vi "From JSON.vi"(8 "error in (no error)":errorcluster, 11 "JSON":string) -> (0 "error out":errorcluster, 3 "Package out":refnum<class "Package.lvclass">)   [LabVIEW 2020, in "GCentral-API.lvlib" / "Package.lvclass"]
uses:
  Package.lvclass
  Package.lvclass/Package.ctl
  neg-pkg/JSON/JSON.lvlib
  Version/Version.lvclass
  Developer Group/Developer Group.lvclass
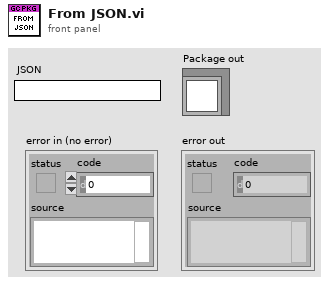
[diagram p1: front panel]
types:
  T1 = typedef "JSON.lvlib/JSON Item Type.ctl" = enum16{"unknown", "null", "Array", "Object", "String", "Number", "Boolean"}
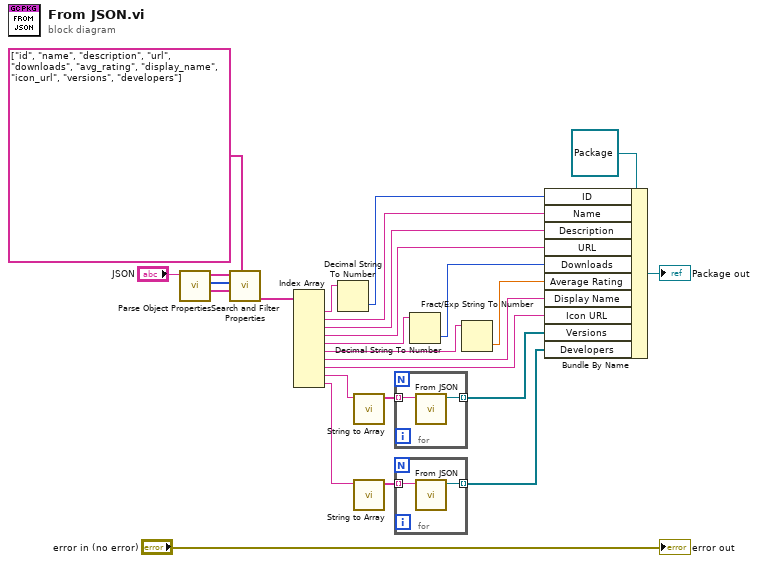
[diagram p0: block diagram]
diagram:
  n1 = call "Parse Object Properties.vi"("JSON String"="JSON") -> ("Values"=w20:string[], "Item Types"=w21:T1[], "Keys"=w22:string[])  [unwired: 7 in, 1 out]
  n2 = call "Search and Filter Properties.vi"("Search Keys"=string[] ["id", "name", "description", "url", "downloads", "avg_rating", "display_name", "icon_url", "versions", "developers"], "Values In"=w20, "Types In"=w21, "Keys In"=w22) -> ("Filtered Values"=w1:string[])  [unwired: 2 in, 5 out]
  n3 = Index Array(array=w1) -> (element #1=w18:string, element #2=w16:string, element #3=w15:string, element #4=w14:string, element #5=w13:string, element #6=w11:string, element #7=w9:string, element #8=w8:string, element #9=w7:string, element #10=w6:string)  [unwired: 10 in]
  n4 = Decimal String To Number(string=w18) -> (number=w17:i32)  [unwired: 2 in, 1 out]
  n5 = call "String to Array.vi"("Array String In"=w7) -> ("JSON Strings"=w5:string[])  [unwired: 10 in]
  n6 = call "String to Array.vi"("Array String In"=w6) -> ("JSON Strings"=w3:string[])  [unwired: 10 in]
  n7 = for {
    tunnel: w5 -> [w28] mode=indexing
    tunnel: [w27] -> w4 mode=indexing
    n8 = call "From JSON.vi"("JSON"=w28) -> ("Version"=w27:refnum<class "Version.lvclass">)  [unwired: 9 in, 1 out]
  }
  n9 = for {
    tunnel: w3 -> [w30] mode=indexing
    tunnel: [w29] -> w2 mode=indexing
    n10 = call "From JSON.vi"("JSON"=w30) -> ("Developer Group out"=w29:refnum<class "Developer Group.lvclass">)  [unwired: 9 in, 1 out]
  }
  n11 = Decimal String To Number(string=w13) -> (number=w12:i32)  [unwired: 2 in, 1 out]
  n12 = Fract/Exp String To Number(string=w11) -> (number=w10:dbl)  [unwired: 3 in, 1 out]
  n13 = Bundle By Name(cluster=refnum<class "Package.lvclass"> refnum ("GCentral-API.lvlib:Package.lvclass"), "ID"=w17, "Name"=w16, "Description"=w15, "URL"=w14, "Downloads"=w12, "Average Rating"=w10, "Display Name"=w9, "Icon URL"=w8, "Versions"=w4, "Developers"=w2) -> (→"Package out":refnum<class "Package.lvclass">)
  "error out" <- "error in (no error)"
